vi "Begin.vi"(11 "Image Size":T1=enum."160x120") -> (0 "error out":errorcluster)   [LabVIEW 2012]
doc: "Called before other user functions, this VI is expected to open initial I/O refnums, load in file data, and do all program initialization. Notice that the <B>error out</B> terminal is simply used for data flow. Wiring it to other structures or subVIs ensures that this VI runs first."
uses:
  <vilib>/Rock Robotics/WPI/Camera/WPI_CameraImageSize.ctl
  <vilib>/Rock Robotics/WPI/Camera/WPI_CameraWhite Balance Values.ctl
  <vilib>/Rock Robotics/WPI/Camera/WPI_CameraExposure Values.ctl
  <vilib>/Rock Robotics/WPI/Camera/WPI_CameraFrameRate.ctl
  <vilib>/Rock Robotics/WPI/DriverStation/WPI_DriverStationRobotMode2.ctl
  <vilib>/Rock Robotics/WPI/Joystick/WPI_JoystickDeviceEnum.ctl
  <vilib>/Rock Robotics/SystemInterfaces/DIO/FPGA_DIOPWMChannel.ctl
  <vilib>/Rock Robotics/WPI/SafetyOutput/WPI_SafetyOutputConfigMenu.ctl
  <vilib>/Rock Robotics/SystemInterfaces/DIO/FPGA_DIORelayChannel.ctl
  Robot Global Data.vi
  <vilib>/Rock Robotics/WPI/MotorControl/WPI_MotorControlOpen Jaguar.vi
  <vilib>/Rock Robotics/WPI/RobotDrive/WPI_RobotDriveOpen2MotorWithJaguar.vi
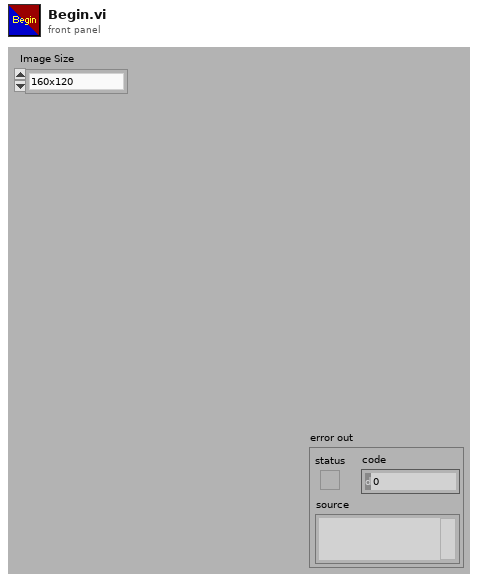
[diagram p1: front panel]
types:
  T1 = typedef "WPI_CameraImageSize.ctl" = enum16{"640x480", "320x240", "160x120"}
  T2 = typedef "FPGA_DIORelayChannel.ctl" = enum8{"Relay 1", "Relay 2", "Relay 3", "Relay 4", "Relay 5", "Relay 6", "Relay 7", "Relay 8", "Invalid"}
  T3 = typedef "WPI_SafetyOutputConfigMenu.ctl" = enum16{"Enable", "Disable"}
  T4 = typedef "FPGA_DIOPWMChannel.ctl" = enum8{"PWM 1", "PWM 2", "PWM 3", "PWM 4", "PWM 5", "PWM 6", "PWM 7", "PWM 8", "PWM 9", "PWM 10", "Invalid"}
  T5 = typedef "WPI_JoystickDeviceEnum.ctl" = enum16{"USB 1", "USB 2", "USB 3", "USB 4", "Kinect 1", "Kinect 2"}
  T6 = typedef "WPI_DriverStationRobotMode2.ctl" = enum16{"Autonomous Disabled", "Autonomous Enabled", "Teleop Disabled", "Teleop Enabled", "Timeout", "Finish", "Test Disabled", "Test Enabled"}
  T7 = typedef "WPI_CameraFrameRate.ctl" = u32
  T8 = typedef "WPI_CameraExposure Values.ctl" = enum16{"Auto", "Flicker-free 50 Hz", "Flicker-free 60 Hz", "Hold current"}
  T9 = typedef "WPI_CameraWhite Balance Values.ctl" = enum16{"Auto", "Fixed indoor", "Fixed outdoor 1", "Fixed outdoor 2", "Fixed fluorescent 1", "Fixed fluorescent 2", "Hold current"}
  T10 = typedef "WPI_JoystickDevRef.ctl" = cluster{"Device":T5}
  T11 = typedef "WPI_RelayDevRef.ctl" = cluster{"DevStatus":errorcluster, "Relay Channel":T2, "Digital Module":T12, "Relay Direction":T13}
  T12 = typedef "FPGA_TypedefDigitalModule.ctl" = enum16{"Digital Module 1", "Digital Module 2"}
  T13 = typedef "WPI_RelayDirection.ctl" = enum16{"Both directions", "Forward only", "Reverse only"}
  T14 = typedef "WPI_MotorControlDeviceRef.ctl" = cluster{"DeviceStatus":errorcluster, "Type":enum16{"PWM", "CAN"}, "PWM":cluster{"Digital Module":T12, "PWM Channel":T4, "DeadBand":T15}, "CAN":cluster{"Device Number":u8, "Control Mode":T16, "Semaphore":T17, "Max Vout":dbl}, "Invert":bool, "TransformRef":T18, "InvTransformRef":T18}
  T15 = typedef "WPI_PWMDeadband.ctl" = cluster{"Name":string, "maxPositivePwm":i32, "minPositivePwm":i32, "centerPwm":i32, "maxNegativePwm":i32, "minNegativePwm":i32, "angularRange":u16}
  T16 = typedef "WPI_CANJaguar_ControlMode.ctl" = enum8{"Percent VBus", "Current", "Speed", "Position", "Voltage"}
  T17 = typedef "Semaphore RefNum" = refnum<k1>
  T18 = typedef "WPI_PWMTransform_ConPane.ctl" = refnum<vi>
  T19 = typedef "WPI_RobotDriveDevRef.ctl" = cluster{"DevStatus":errorcluster, "Motors[]":T14[], "Square Inputs":bool, "Max Output":dbl, "Isochronous":bool}
  T20 = typedef "WPI_CameraDevRef.ctl" = cluster{"Camera Address":string, "CameraStatus":errorcluster, "Acquire Image Notifier":refnum<notifier>}
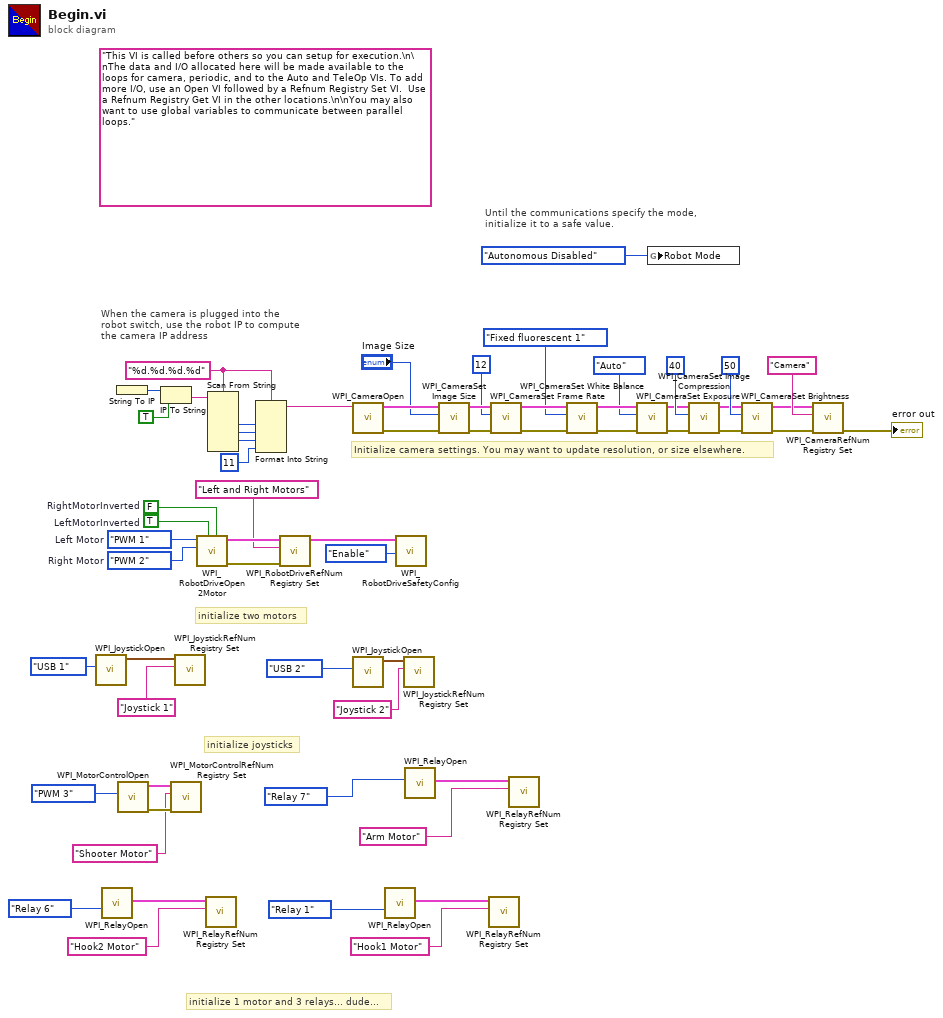
[diagram p0: block diagram]
diagram:
  w11 = FPGA_DIOPWMChannel."PWM 2"  # Right Motor
  w12 = FPGA_DIOPWMChannel."PWM 1"  # Left Motor
  w16 = TRUE  # LeftMotorInverted
  w17 = FALSE  # RightMotorInverted
  w32 = "%d.%d.%d.%d" ("format string")
  (unwired) "This VI is called before others so you can setup for execution.\n\nThe data and I/O allocated here will be made available to the loops for camera, periodic, and to the Auto and TeleOp VIs. To add more I/O, use an Open VI followed by a Refnum Registry Set VI.  Use a Refnum Registry Get VI in the other locations.\n\nYou may also want to use global variables to communicate between parallel loops."
  # "initialize two motors"
  # "initialize 1 motor and 3 relays... dude..."
  # "initialize joysticks"
  # "Until the communications specify the mode,\ninitialize it to a safe value."
  # "When the camera is plugged into the\nrobot switch, use the robot IP to compute\nthe camera IP address"
  # "Initialize camera settings. You may want to update resolution, or size elsewhere."
  n1 = call <vilib>:"WPI_JoystickOpen.vi"("JoystickDevice"=WPI_JoystickDeviceEnum."USB 1") -> ("JoystickDevRef"=w27:T10)  [unwired: 10 in]
  n2 = call <vilib>:"WPI_RelayOpen.vi"("Relay Channel"=FPGA_DIORelayChannel."Relay 6") -> ("RelayDevRef"=w8:T11)  [unwired: 9 in, 1 out]
  n3 = String To IP() -> (0:w39:u32)  [unwired: 1 in]
  n4 = call-poly <vilib>:"WPI_MotorControlOpen.vi"("PWM Channel"=FPGA_DIOPWMChannel."PWM 3") -> ("error out"=w21:errorcluster, "MotorControlDeviceRef"=w22:T14)  [unwired: 9 in]
  n5 = IP To String(1:TRUE ("dot notation? (F)"), 2:w39) -> (0:w37:string)
  n6 = call <vilib>:"WPI_MotorControlRefNum Registry Set.vi"("error in (no error)"=w21, "refnum name"="Shooter Motor", "MotorControlDevRef"=w22) -> ()  [unwired: 7 in, 2 out]
  n7 = call <vilib>:"WPI_JoystickRefNum Registry Set.vi"("refnum name"="Joystick 1", "JoystickDevRef"=w27) -> ()  [unwired: 8 in, 2 out]
  n8 = call-poly <vilib>:"WPI_RobotDriveOpen2Motor.vi"("Right Motor Inverted"=w17, "Left Motor Inverted"=w16, "Right Motor"=w11, "Left Motor"=w12) -> ("error out"=w13:errorcluster, "RobotDriveDevRef"=w15:T19)  [unwired: 6 in]
  n9 = call <vilib>:"WPI_RelayRefNum Registry Set.vi"("refnum name"="Hook2 Motor", "RelayDevRef"=w8) -> ()  [unwired: 8 in, 2 out]
  n10 = Scan From String(format string=w32, input string=w37) -> (output 1=w36:i32, output 2=w35:i32, output 3=w34:i32)  [unwired: 7 in, 3 out]
  n11 = Format Into String(format string=w32, w36, w35, w34, 11 ("Compression")) -> (resulting string=w30:string)  [unwired: 2 in, 1 out]
  n12 = call <vilib>:"WPI_RobotDriveRefNum Registry Set.vi"("error in (no error)"=w13, "refnum name"="Left and Right Motors", "RobotDriveDevRef"=w15) -> ("RobotDriveDevRef"=w10:T19)  [unwired: 8 out]
  n13 = call <vilib>:"WPI_CameraOpen.vi"("Camera Address"=w30) -> ("error out"=w51:errorcluster, "CameraDevRef"=w52:T20)  [unwired: 1 in, 8 out]
  n14 = call <vilib>:"WPI_JoystickOpen.vi"("JoystickDevice"=WPI_JoystickDeviceEnum."USB 2") -> ("JoystickDevRef"=w25:T10)  [unwired: 10 out]
  n15 = call <vilib>:"WPI_RelayOpen.vi"("Relay Channel"=FPGA_DIORelayChannel."Relay 1") -> ("RelayDevRef"=w5:T11)  [unwired: 9 in, 1 out]
  n16 = call <vilib>:"WPI_RobotDriveSafetyConfig.vi"("mode"=WPI_SafetyOutputConfigMenu."Enable", "RobotDriveDevRef"=w10) -> ()  [unwired: 8 in, 2 out]
  n17 = call <vilib>:"WPI_JoystickRefNum Registry Set.vi"("refnum name"="Joystick 2", "JoystickDevRef"=w25) -> ()  [unwired: 1 in, 9 out]
  n18 = call <vilib>:"WPI_RelayOpen.vi"("Relay Channel"=FPGA_DIORelayChannel."Relay 7") -> ("RelayDevRef"=w3:T11)  [unwired: 9 in, 1 out]
  n19 = call <vilib>:"WPI_CameraSet Image Size.vi"("error in (no error)"=w51, "Image Size"="Image Size", "CameraDevRef"=w52) -> ("error out"=w50:errorcluster, "CameraDevRef Out"=w53:T20)  [unwired: 7 out]
  n20 = call <vilib>:"WPI_RelayRefNum Registry Set.vi"("refnum name"="Hook1 Motor", "RelayDevRef"=w5) -> ()  [unwired: 8 in, 2 out]
  n21 = call <vilib>:"WPI_CameraSet Frame Rate.vi"("error in (no error)"=w50, "Frame Rate (fps)"=T7 12, "CameraDevRef"=w53) -> ("error out"=w49:errorcluster, "CameraDevRef Out"=w55:T20)  [unwired: 7 out]
  n22 = call <vilib>:"WPI_RelayRefNum Registry Set.vi"("refnum name"="Arm Motor", "RelayDevRef"=w3) -> ()  [unwired: 8 in, 2 out]
  n23 = call <vilib>:"WPI_CameraSet White Balance.vi"("error in (no error)"=w49, "White Balance"=WPI_CameraWhite_Balance_Values."Fixed fluorescent 1", "CameraDevRef"=w55) -> ("error out"=w48:errorcluster, "CameraDevRef Out"=w54:T20)  [unwired: 7 out]
  n24 = call <vilib>:"WPI_CameraSet Exposure.vi"("error in (no error)"=w48, "Exposure"=WPI_CameraExposure_Values."Auto", "CameraDevRef"=w54) -> ("error out"=w47:errorcluster, "CameraDevRef Out"=w57:T20)  [unwired: 7 out]
  n25 = global write "Robot Global Data.vi" "Robot Mode"(WPI_DriverStationRobotMode2."Autonomous Disabled" ("Robot Mode")) -> ()
  n26 = call <vilib>:"WPI_CameraSet Image Compression.vi"("error in (no error)"=w47, "Compression"=40, "CameraDevRef"=w57) -> ("error out"=w46:errorcluster, "CameraDevRef Out"=w56:T20)  [unwired: 7 out]
  n27 = call <vilib>:"WPI_CameraSet Brightness.vi"("error in (no error)"=w46, "Brightness"=50, "CameraDevRef"=w56) -> ("error out"=w44:errorcluster, "CameraDevRef Out"=w45:T20)  [unwired: 7 out]
  n28 = call <vilib>:"WPI_CameraRefNum Registry Set.vi"("error in (no error)"=w44, "refnum name"="Camera", "CameraDevRef"=w45) -> ("error out"=→"error out":errorcluster)  [unwired: 8 out]
